vi "pad_sensitivity.vi"(9 "input variable":i8) -> (1 "output variable":i8)   [LabVIEW 2012]
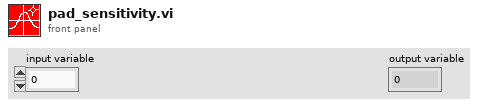
[diagram p1: front panel]
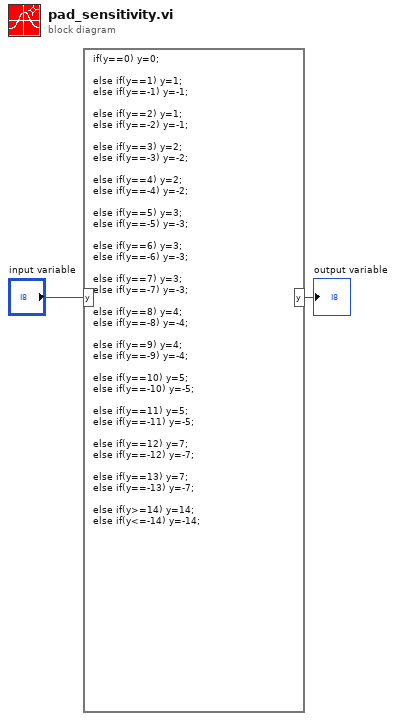
[diagram p0: block diagram]
diagram:
  n1 = formula code="if(y==0) y=0;\n\nelse if(y==1) y=1;\nelse if(y==-1) y=-1;\n\nelse if(y==2) y=1;\nelse if(y==-2) y=-1;\n\nelse if(y==3) y=2;\nelse if(y==-3) y=-2;\n\nelse if(y==4) y=2;\nelse if(y==-4) y=-2;\n\nelse if(y==5) y=3;\nelse if(y==-5) y=-3;\n\nelse if(y==6) y=3;\nelse if(y==-6) y=-3;\n\nelse if(y==7) y=3;\nelse if(y==-7) y=-3;\n\nelse if(y==8) y=4;\nelse if(y==-8) y=-4;\n\nelse if(y==9) y=4;\nelse if(y==-9) y=-4;\n\nelse if(y==10) y=5;\nelse if(y==-10) y=-5;\n\nelse if(y==11) y=5;\nelse if(y==-11) y=-5;\n\nelse if(y==12) y=7;\nelse if(y==-12) y=-7;\n\nelse if(y==13) y=7;\nelse if(y==-13) y=-7;\n\nelse if(y>=14) y=14; \nelse if(y<=-14) y=-14;"("y"="input variable") -> ("y"=→"output variable":i8)
